vi "FusePose.vi"(2 "Pose Mode":T1(ring), 5 "Vision Trust Threshold (in)":dbl, 7 "Vision Valid [t-?]":bool, 8 "Odometry Delta Y (in) [t0]":dbl, 9 "Vision Y (in) [t-?]":dbl, 10 "Odometry Delta X (in) [t0]":dbl, 11 "Vision X (in) [t-?]":dbl, 12 "Odometry Timestamp (ms)":u32, 13 "Vision Timestamp (ms)":u32) -> (14 "X (in) [t0]":dbl, 15 "Y (in) [t0]":dbl)   [LabVIEW 2020]
doc: "This VI fuses multiple sensing modalities to estimate the robot's current pose."
uses:
  <vilib>/Rock Robotics/WPI/DriverStation/WPI_DriverStationRobotMode2.ctl
  61fa55d1-284c-4213-a227-888cd534c963.vi
  b35b41c9-1c56-41de-b07f-09edca4c47f7.vi
  7b9bb9b1-306e-4d3e-b7ed-2eba6d8170c6.vi
  1559d662-8abd-40e9-a5dc-3c53134ee71a.vi
  524daecc-998c-4826-9d6e-2db19cf0bc7c.vi
  robotconstants.vi
  driverdata.vi
  autonomousinfo.vi
  sensordata.vi
  <vilib>/Analysis/NI_AALBase.lvlib
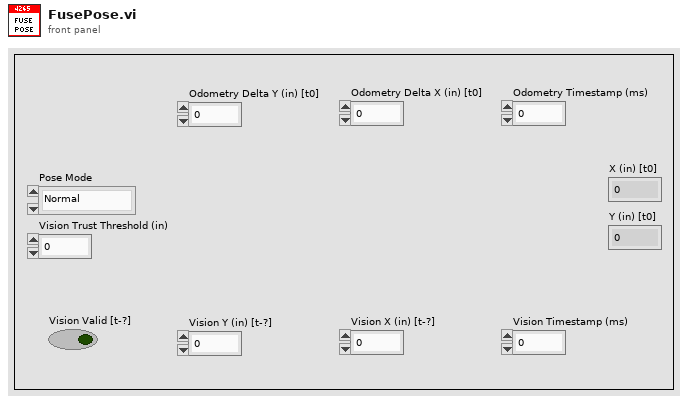
[diagram p1: front panel]
types:
  T1 = enum16{"Normal", "Auto Set", "Reset IMU", "Manual Push", "Init"}
  T2 = typedef "WPI_DriverStationRobotMode2.ctl" = enum16{"Autonomous Disabled", "Autonomous Enabled", "Teleop Disabled", "Teleop Enabled", "Disconnected", "Finish", "Test Disabled", "Test Enabled", "Emergency Stopped"}
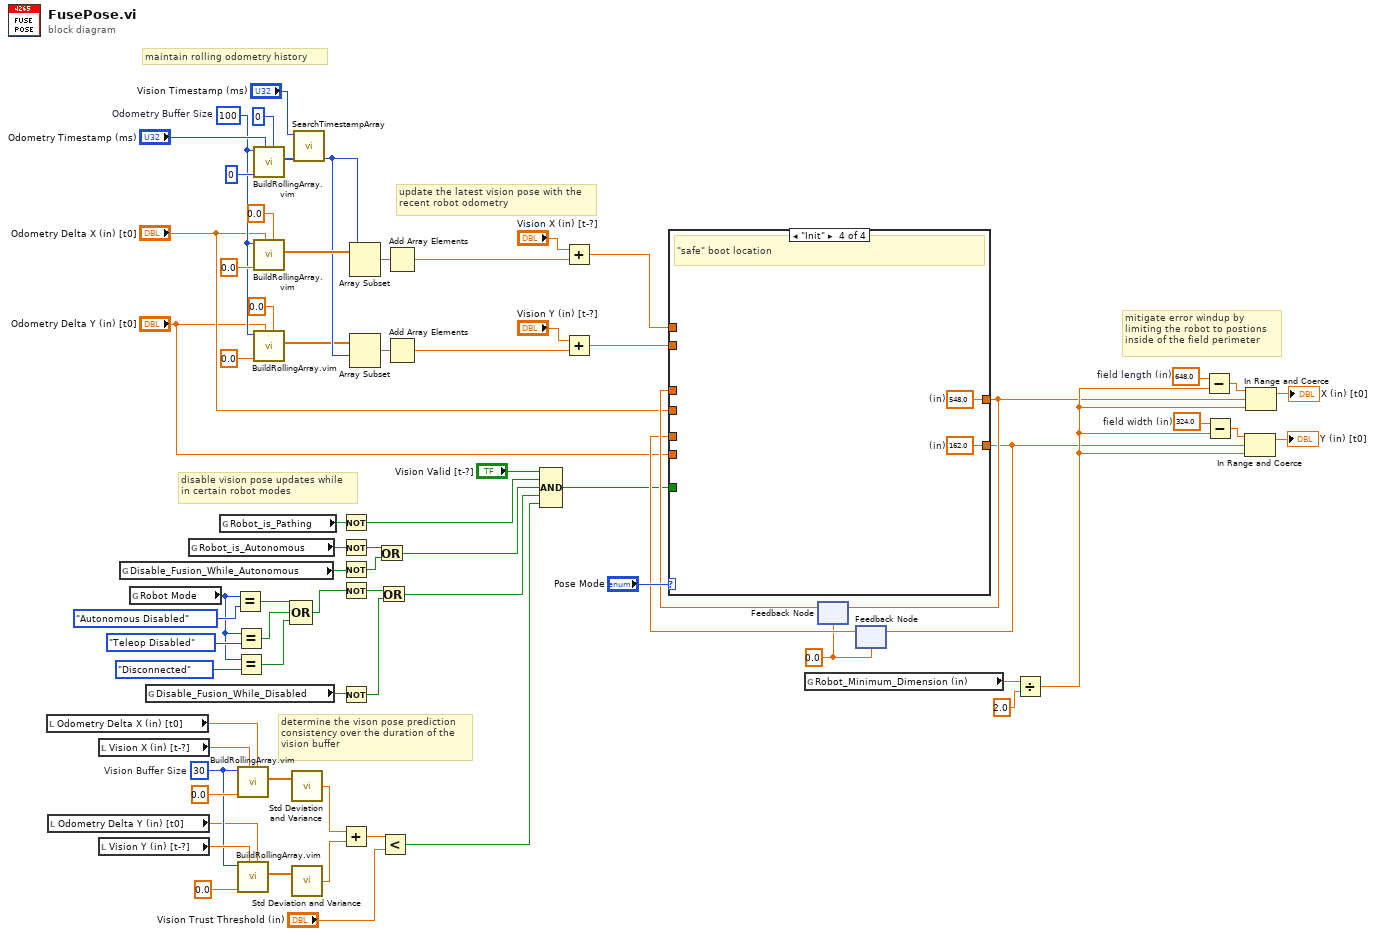
[diagram p0: block diagram]
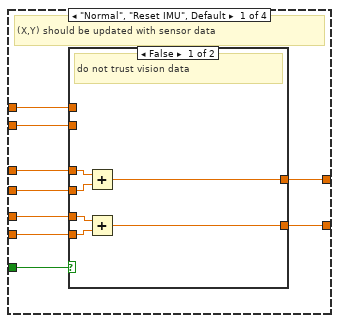
[diagram p2: hidden frame]
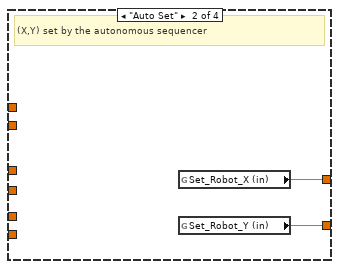
[diagram p4: hidden frame]
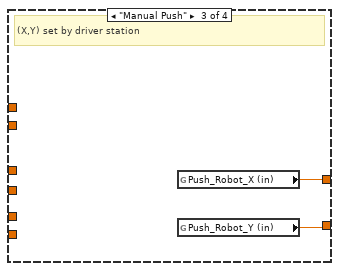
[diagram p5: hidden frame]
diagram:
  w32 = 30  # Vision Buffer Size
  w45 = 0.0
  w53 = 648.0  # field length (in)
  w54 = 324.0  # field width (in)
  w40 = 100  # Odometry Buffer Size
  # "disable vision pose updates while\nin certain robot modes"
  # "determine the vison pose prediction\nconsistency over the duration of the\nvision buffer"
  # "maintain rolling odometry history"
  # "update the latest vision pose with the\nrecent robot odometry"
  # "mitigate error windup by\nlimiting the robot to postions\ninside of the field perimeter"
  n1 = local read "Odometry Delta X (in) [t0]"() -> (w30:dbl)
  n2 = local read "Odometry Delta Y (in) [t0]"() -> (w29:dbl)
  n3 = local read "Vision X (in) [t-?]"() -> (w34:dbl)
  n4 = local read "Vision Y (in) [t-?]"() -> (w33:dbl)
  n5 = global read "driverdata.vi" "Disable_Fusion_While_Autonomous"() -> (w15:bool)
  n6 = global read "driverdata.vi" "Robot Mode"() -> (w3:T2)
  n7 = global read "driverdata.vi" "Disable_Fusion_While_Disabled"() -> (w21:bool)
  n8 = global read "driverdata.vi" "Robot_is_Autonomous"() -> (w17:bool)
  n9 = global read "autonomousinfo.vi" "Robot_is_Pathing"() -> (w19:bool)
  n10 = Equal?(x=w3, y=WPI_DriverStationRobotMode2."Autonomous Disabled" ("Robot Mode")) -> (x = y?=w8:bool)
  n11 = Equal?(x=w3, y=WPI_DriverStationRobotMode2."Teleop Disabled") -> (x = y?=w6:bool)
  n12 = Equal?(x=w3, y=WPI_DriverStationRobotMode2."Disconnected") -> (x = y?=w1:bool)
  n13 = call "BuildRollingArray.vim"("Global Additive Update"=w30, "New Value"=w34, "Initial Value"=0.0, "Number of Elements"=w32) -> ("Current Array"=w28:dbl[])  [unwired: 7 in]
  n14 = call "BuildRollingArray.vim"("Global Additive Update"=w29, "New Value"=w33, "Initial Value"=0.0, "Number of Elements"=w32) -> ("Current Array"=w27:dbl[])  [unwired: 7 in]
  n15 = call "BuildRollingArray.vim"("Global Additive Update"=0, "New Value"="Odometry Timestamp (ms)", "Initial Value"=0, "Number of Elements"=w40) -> ("Current Array"=w69:u32[])  [unwired: 7 in]
  n16 = call "BuildRollingArray.vim"("Global Additive Update"=0.0, "New Value"="Odometry Delta X (in) [t0]", "Initial Value"=0.0, "Number of Elements"=w40) -> ("Current Array"=w66:dbl[])  [unwired: 7 in]
  n17 = call "BuildRollingArray.vim"("Global Additive Update"=0.0, "New Value"="Odometry Delta Y (in) [t0]", "Initial Value"=0.0, "Number of Elements"=w40) -> ("Current Array"=w61:dbl[])  [unwired: 7 in]
  n18 = Compound Arithmetic op=OR(w8, w6, w1) -> (w7:bool)
  n19 = call <vilib>:"Std Deviation and Variance.vi"("X"=w28) -> ("standard deviation"=w26:dbl)  [unwired: 1 in, 2 out]
  n20 = call <vilib>:"Std Deviation and Variance.vi"("X"=w27) -> ("standard deviation"=w25:dbl)  [unwired: 1 in, 2 out]
  n21 = call "SearchTimestampArray.vi"("Timestamp Array"=w69, "Search Timestamp"="Vision Timestamp (ms)") -> ("Closest Index"=w62:i32)  [unwired: 8 in, 1 out]
  n22 = Not(x=w19) -> (.not. x?=w18:bool)
  n23 = Not(x=w17) -> (.not. x?=w16:bool)
  n24 = Not(x=w15) -> (.not. x?=w14:bool)
  n25 = Not(x=w7) -> (.not. x?=w10:bool)
  n26 = Not(x=w21) -> (.not. x?=w11:bool)
  n27 = Add(x=w26, y=w25) -> (x+y=w24:dbl)
  n28 = Array Subset(array=w66, index=w62) -> (w67:dbl[])  [unwired: 1 in]
  n29 = Array Subset(array=w61, index=w62) -> (w64:dbl[])  [unwired: 1 in]
  n30 = Or(x=w16, y=w14) -> (x .or. y?=w12:bool)
  n31 = Or(x=w10, y=w11) -> (x .or. y?=w9:bool)
  n32 = Less?(x=w24, y="Vision Trust Threshold (in)") -> (x < y?=w13:bool)
  n33 = Add Array Elements(numeric array=w67) -> (sum=w65:dbl)
  n34 = Add Array Elements(numeric array=w64) -> (sum=w63:dbl)
  n35 = Compound Arithmetic op=AND("Vision Valid [t-?]", w18, w12, w9, w13) -> (w22:bool)
  n36 = Add(x="Vision X (in) [t-?]", y=w65) -> (x+y=w58:dbl)
  n37 = Add(x="Vision Y (in) [t-?]", y=w63) -> (x+y=w59:dbl)
  n38 = global read "robotconstants.vi" "Robot_Minimum_Dimension (in)"() -> (w57:dbl)
  n39 = feedback #1(w45) -> (w48:dbl)
  n40 = feedback #2(w45) -> (w46:dbl)
  n41 = case shown="\"Init\"" "Pose Mode" {
    tunnel: [w78 w92 w94 w96] -> w49
    tunnel: w48 -> [w82 _ _ _]
    tunnel: "Odometry Delta X (in) [t0]" -> [w81 _ _ _]
    tunnel: w46 -> [w80 _ _ _]
    tunnel: "Odometry Delta Y (in) [t0]" -> [w79 _ _ _]
    tunnel: [w77 w91 w93 w95] -> w47
    tunnel: w22 -> [w76 _ _ _]
    tunnel: w59 -> [w75 _ _ _]
    tunnel: w58 -> [w74 _ _ _]
    frame "Normal", "Reset IMU", Default {
      # "(X,Y) should be updated with sensor data"
      n42 = case shown="False" w76 {
        tunnel: w82 -> [w87 _]
        tunnel: w81 -> [w88 _]
        tunnel: w80 -> [w86 _]
        tunnel: w79 -> [w85 _]
        tunnel: [w84 w89] -> w78
        tunnel: [w83 w90] -> w77
        tunnel: w75 -> [_ w90]
        tunnel: w74 -> [_ w89]
        frame False {
          # "do not trust vision data"
          n43 = Add(x=w87, y=w88) -> (x+y=w84:dbl)
          n44 = Add(x=w86, y=w85) -> (x+y=w83:dbl)
        }
        frame True {
          # "trust vision data"
        }
      }
    }
    frame "Auto Set" {
      # "(X,Y) set by the autonomous sequencer"
      n45 = global read "sensordata.vi" "Set_Robot_X (in)"() -> (w92:dbl)
      n46 = global read "sensordata.vi" "Set_Robot_Y (in)"() -> (w91:dbl)
    }
    frame "Manual Push" {
      # "(X,Y) set by driver station"
      n47 = global read "sensordata.vi" "Push_Robot_X (in)"() -> (w94:dbl)
      n48 = global read "sensordata.vi" "Push_Robot_Y (in)"() -> (w93:dbl)
    }
    frame "Init" {
      w95 = 162.0  # (in)
      w96 = 548.0  # (in)
      # "\"safe\" boot location"
    }
  }
  n49 = feedback-in #1(w49) -> ()
  n50 = feedback-in #2(w47) -> ()
  n51 = Divide(x=w57, y=2.0) -> (x/y=w52:dbl)
  n52 = Subtract(x=w53, y=w52) -> (x-y=w51:dbl)
  n53 = Subtract(x=w54, y=w52) -> (x-y=w55:dbl)
  n54 = In Range and Coerce(upper limit=w55, x=w47, lower limit=w52) -> (coerced(x)=→"Y (in) [t0]":dbl)  [unwired: 1 out]
  n55 = In Range and Coerce(upper limit=w51, x=w49, lower limit=w52) -> (coerced(x)=→"X (in) [t0]":dbl)  [unwired: 1 out]
